vi "Get Available Port.vi"(7 "net address":u32) -> (8 "port":u16, 15 "error out":errorcluster)   [LabVIEW 2020, in "epl-network.lvlib"]
uses:
  epl-network.lvlib
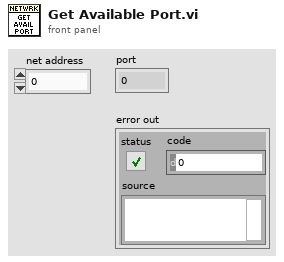
[diagram p1: front panel]
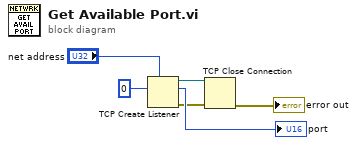
[diagram p0: block diagram]
diagram:
  n1 = TCP Create Listener(7:"net address", 10:u16 0 ("port")) -> (0:w2:errorcluster, 2:→"port":u16, 3:w3:refnum<k5>)  [unwired: 3 in]
  n2 = TCP Close Connection(connection ID=w3, error in (no error)=w2) -> (error out=→"error out":errorcluster)  [unwired: 1 in, 1 out]
